vi "parseHP.vi"(8 "error in (no error)":errorcluster, 10 "ModbusBuffer in":refnum<class "ModbusBuffer.lvclass">, 11 "HPILC in":refnum<class "HPILC.lvclass">) -> (0 "error out":errorcluster, 1 "ParseSuccessful":bool, 2 "ModbusBuffer out":refnum<class "ModbusBuffer.lvclass">, 3 "HPILC out":refnum<class "HPILC.lvclass">)   [LabVIEW 2016, in "RTHPILC.lvlib" / "HPILC.lvclass"]
uses:
  HPILC.lvclass
  D:/Code/ts_M1M3Support/Common_RT_ILC/ILC/ILC.lvclass
  Common_RT_Modbus/ModbusBuffer/ModbusBuffer.lvclass
  Common_RT_Modbus/ModbusBuffer/ModbusBuffer.lvclass/ModbusBuffer.ctl
  Common_RT_ILC/ILC/ILC.lvclass/ILC.ctl
  HPILC.lvclass/HPILC.ctl
  Common_RT_ILC/ILC/parseReportServerIDFrame.vi
  Common_RT_ILC/ILC/parseReportServerIDError.vi
  Common_RT_ILC/ILC/parseReportServerStatusFrame.vi
  Common_RT_ILC/ILC/parseReportServerStatusError.vi
  Common_RT_ILC/ILC/parseModeFrame.vi
  Common_RT_ILC/ILC/parseModeError.vi
  Common_RT_ILC/ILC/parseTemporaryAddressFrame.vi
  Common_RT_ILC/ILC/parseTemporaryAddressError.vi
  Common_RT_ILC/ILC/parseADCScanRateFrame.vi
  Common_RT_ILC/ILC/parseADCScanRateError.vi
  Common_RT_ILC/ILC/parseADCOffsetSensitivityFrame.vi
  Common_RT_ILC/ILC/parseADCOffsetSensitivityError.vi
  Common_RT_ILC/ILC/parseResetFrame.vi
  Common_RT_ILC/ILC/parseResetError.vi
  Common_RT_ILC/ILC/parseReportCalibrationDataFrame.vi
  Common_RT_ILC/ILC/parseReportCalibrationDataError.vi
  Common_RT_Modbus/ModbusBuffer/calculateCRC.vi
  Common_RT_Modbus/ModbusBuffer/readCRC.vi
  Common_RT_Modbus/ModbusBuffer/readTimestamp.vi
  Common_RT_Modbus/ModbusBuffer/readEndOfFrame.vi
  Common_RT_Modbus/ModbusBuffer/readI32.vi
  Common_RT_Modbus/ModbusBuffer/readSGL.vi
  Common_RT_Modbus/ModbusBuffer/readInstructionByte.vi
  Common_RT_Modbus/ModbusBuffer/readU48.vi
  Common_RT_Modbus/ModbusBuffer/readString.vi
  Common_RT_Modbus/ModbusBuffer/readU16.vi
  Common_RT_Modbus/ModbusBuffer/readTimestampByte.vi
  Common_RT_ILC/ILC/ILC.lvclass
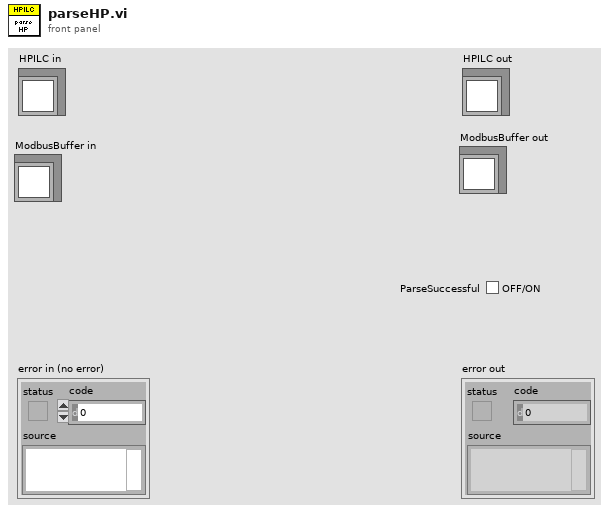
[diagram p1: front panel]
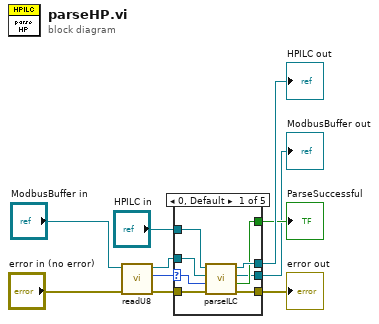
[diagram p0: block diagram]
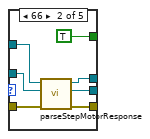
[diagram p2: hidden frame]
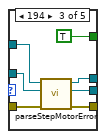
[diagram p3: hidden frame]
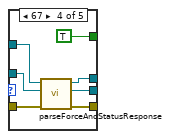
[diagram p4: hidden frame]
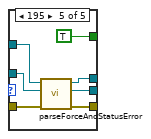
[diagram p5: hidden frame]
diagram:
  n1 = call "readU8.vi"("error in (no error)"="error in (no error)", "ModbusBuffer in"="ModbusBuffer in") -> ("error out"=w4:errorcluster, "Output"=w5:u8, "ModbusBuffer out"=w6:refnum<class "ModbusBuffer.lvclass">)  [unwired: 7 in]
  n2 = case shown="0, Default" w5 {
    selector: w5 -> [w11 _ _ _ _]
    tunnel: w6 -> [w15 w25 w31 w38 w45]
    tunnel: "HPILC in" -> [w18 w24 w32 w39 w46]
    tunnel: [w17 w23 w30 w35 w43] -> w9
    tunnel: [w16 TRUE ("ParseSuccessful") TRUE ("ParseSuccessful") TRUE ("ParseSuccessful") TRUE ("ParseSuccessful")] -> w8
    tunnel: [w13 w22 w28 w37 w44] -> w1
    tunnel: w4 -> [w14 w20 w27 w34 w41]
    tunnel: [w12 w19 w26 w33 w40] -> w2
    frame 0, Default {
      n3 = call "parseILC.vi"("error in (no error)"=w14, "Func"=w11, "ModbusBuffer in"=w15, "ILC in"=w18) -> ("error out"=w13:errorcluster, "ParseSuccessful"=w16:bool, "ModbusBuffer out"=w12:refnum<class "ModbusBuffer.lvclass">, "ILC out"=w17:refnum<class "HPILC.lvclass">)  [unwired: 4 in]
    }
    frame 66 {
      n4 = call "parseStepMotorResponse.vi"("error in (no error)"=w20, "ModbusBuffer in"=w25, "HPILC in"=w24) -> ("error out"=w22:errorcluster, "ModbusBuffer out"=w19:refnum<class "ModbusBuffer.lvclass">, "HPILC out"=w23:refnum<class "HPILC.lvclass">)  [unwired: 6 in]
    }
    frame 194 {
      n5 = call "parseStepMotorError.vi"("error in (no error)"=w27, "ModbusBuffer in"=w31, "HPILC in"=w32) -> ("error out"=w28:errorcluster, "ModbusBuffer out"=w26:refnum<class "ModbusBuffer.lvclass">, "HPILC out"=w30:refnum<class "HPILC.lvclass">)  [unwired: 6 in]
    }
    frame 67 {
      n6 = call "parseForceAndStatusResponse.vi"("error in (no error)"=w34, "ModbusBuffer in"=w38, "HPILC in"=w39) -> ("error out"=w37:errorcluster, "ModbusBuffer out"=w33:refnum<class "ModbusBuffer.lvclass">, "HPILC out"=w35:refnum<class "HPILC.lvclass">)  [unwired: 6 in]
    }
    frame 195 {
      n7 = call "parseForceAndStatusError.vi"("error in (no error)"=w41, "ModbusBuffer in"=w45, "HPILC in"=w46) -> ("error out"=w44:errorcluster, "ModbusBuffer out"=w40:refnum<class "ModbusBuffer.lvclass">, "HPILC out"=w43:refnum<class "HPILC.lvclass">)  [unwired: 6 in]
    }
  }
  "error out" <- w1
  "HPILC out" <- w9
  "ParseSuccessful" <- w8
  "ModbusBuffer out" <- w2
